vi "Module (Top Level).vi"(8 "error in":errorcluster) -> (0 "error out":errorcluster)   [LabVIEW 2017, in "Error Handler.lvlib"]
uses:
  Error Handler.lvlib
  User Events/TypeDefs/Shutdown UE FGV Command.ctl
  Global TypeDefs/Registered Modules.ctl
  <vilib>/Utility/error.llb/DialogType.ctl
  mypam/Public TypeDefs/Module Events.ctl
  Game/Public TypeDefs/Module Events.ctl
  winhost/Public TypeDefs/Module Events.ctl
  Private TypeDefs/Messages.ctl
  Logger/Logger.lvlib
  Controller/Controller.lvlib
  Game/Game.lvlib
  WinHost/WinHost.lvlib
  mypam/myPAM.lvlib
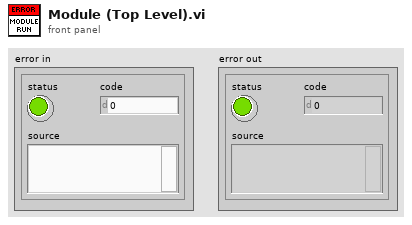
[diagram p1: front panel]
types:
  T1 = typedef "Registered Modules.ctl" = enum16{"Controller", "DAQ", "Error Handler", "Game", "myPAM", "WinHost", "Logger"}
  T2 = typedef "Shutdown UE FGV Command.ctl" = enum16{"create", "get", "destroy"}
  T3 = typedef "Controller.lvlib/Module Reference.ctl" = cluster{"calling module":T1, "module queues":T4, "module notifiers":T5}
  T4 = typedef "Controller.lvlib/Module Queues.ctl" = cluster{"message queue":refnum<queue>}
  T5 = typedef "Controller.lvlib/Module Notifiers.ctl" = cluster{"dummy notifier":refnum<notifier>}
  T6 = typedef "Logger.lvlib/Module Reference.ctl" = cluster{"calling module":T1, "module queues":T7, "module notifiers":T8}
  T7 = typedef "Logger.lvlib/Module Queues.ctl" = cluster{"message queue":refnum<queue>}
  T8 = typedef "Logger.lvlib/Module Notifiers.ctl" = cluster{"dummy notifier":refnum<notifier>}
  T9 = typedef "Error Handler.lvlib/Module Reference.ctl" = cluster{"calling module":T1, "module queues":T10, "module notifiers":T11}
  T10 = typedef "Error Handler.lvlib/Module Queues.ctl" = cluster{"message queue":refnum<queue>}
  T11 = typedef "Error Handler.lvlib/Module Notifiers.ctl" = cluster{"dummy notifier":refnum<notifier>}
  T12 = typedef "myPAM.lvlib/Module Events.ctl" = enum16{"critical error"}
  T13 = typedef "Game.lvlib/Module Events.ctl" = enum16{"client connected", "client status change", "client disconnected"}
  T14 = typedef "WinHost.lvlib/Module Events.ctl" = enum16{"host connected", "enable assistance", "disable assistance", "host disconnected"}
  T15 = typedef "Error Handler.lvlib/Messages.ctl" = enum16{"handle error", "shutdown"}
  T16 = typedef "DialogType.ctl" = u16
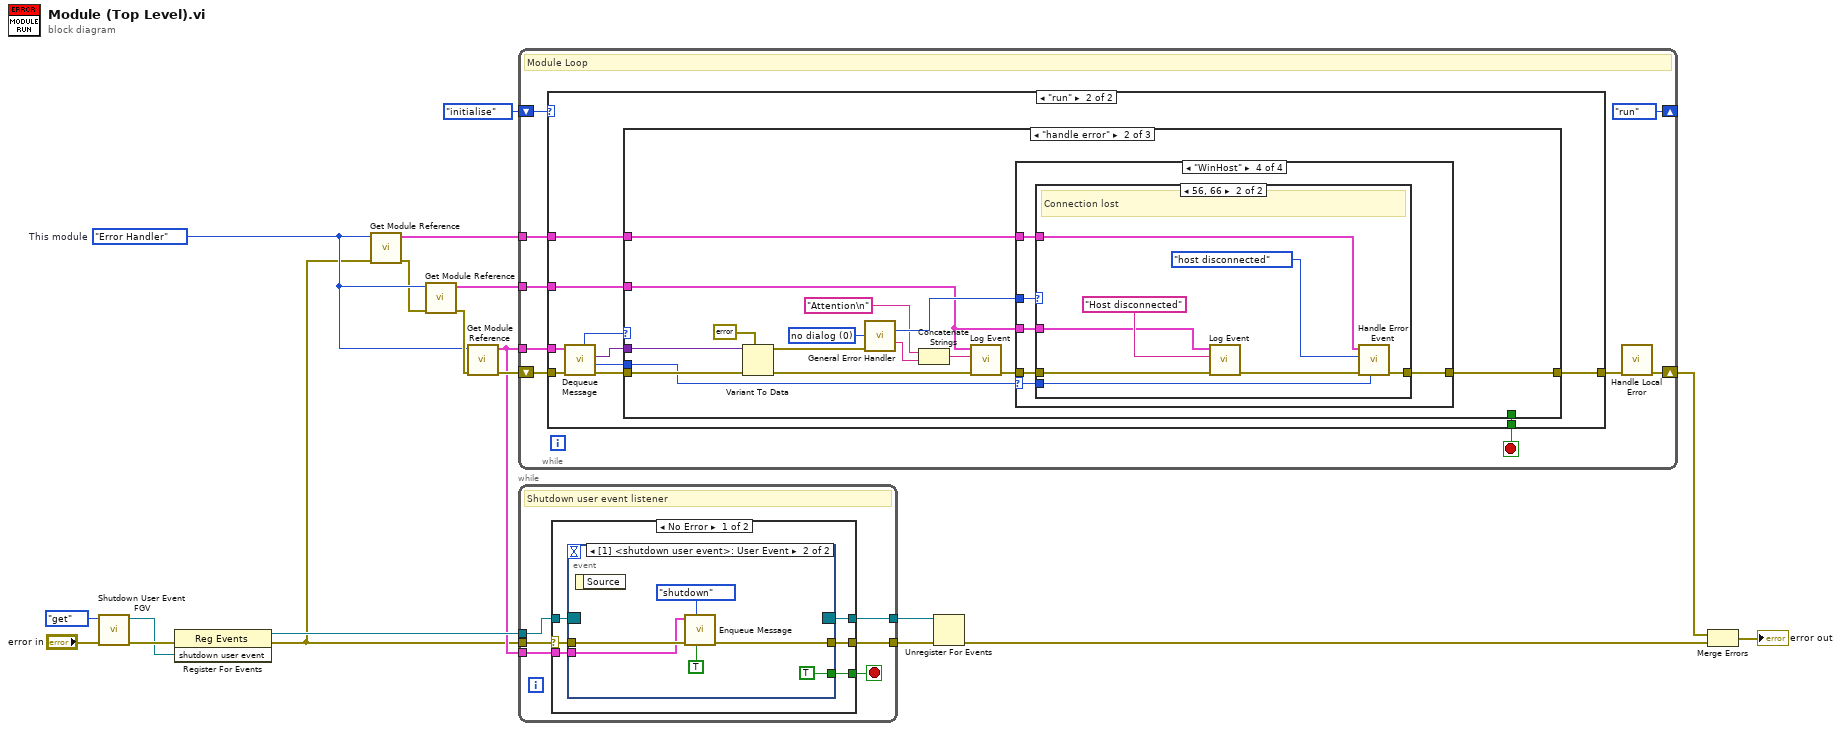
[diagram p0: block diagram]
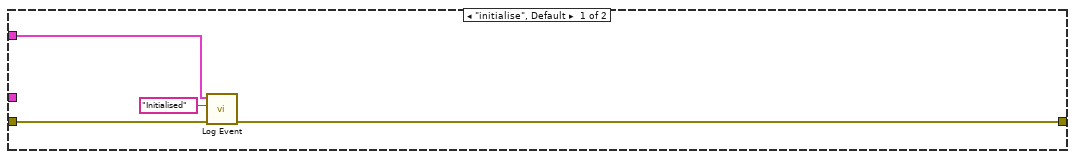
[diagram p2: hidden frame]
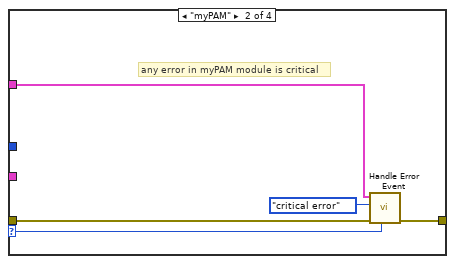
[diagram p5: hidden frame]
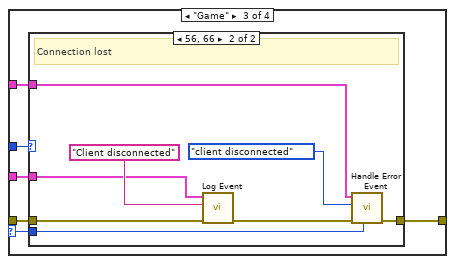
[diagram p6: hidden frame]
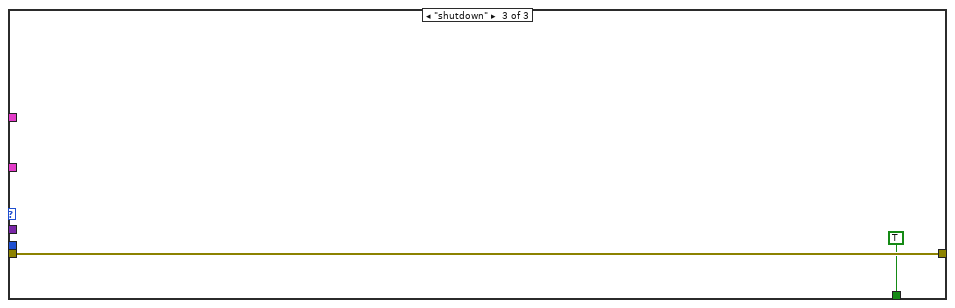
[diagram p9: hidden frame]
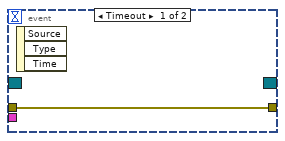
[diagram p10: hidden frame]
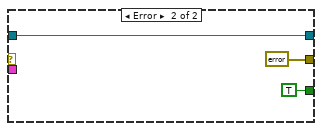
[diagram p11: hidden frame]
diagram:
  w4 = Registered_Modules."Error Handler"  # This module
  n1 = call "Shutdown User Event FGV.vi"("error in"="error in", "command"=Shutdown_UE_FGV_Command."get" ("Command")) -> ("error out"=w14:errorcluster, "shutdown user event"=w13:refnum<user-event>)  [unwired: 8 in]
  n2 = register-events(error in=w14, w13) -> (reference out=w18:refnum<event-registration>, error out=w3:errorcluster)  [unwired: 1 in]
  n3 = call "Get Module Reference.vi"("error in"=w3, "calling module"=w4) -> ("error out"=w2:errorcluster, "module reference"=w1:T3)  [unwired: 8 in]
  n4 = call "Get Module Reference.vi"("error in"=w2, "calling module"=w4) -> ("error out"=w6:errorcluster, "module reference"=w5:T6)  [unwired: 8 in]
  n5 = call "Get Module Reference.vi"("error in"=w6, "calling module"=w4) -> ("error out"=w10:errorcluster, "module reference"=w9:T9)  [unwired: 8 in]
  n6 = while {
    shift-right: [w21] -> w16
    shift-left: w10 -> [w24]
    tunnel: w9 -> [w28]
    shift-right: [enum16{"initialise", "run"}."run"] -> _
    shift-left: enum16{"initialise", "run"}."initialise" -> [w27]
    tunnel: w5 -> [w23]
    tunnel: w1 -> [w20]
    stop <- w25 stop-if-true
    # "Module Loop"
    n7 = case shown="\"run\"" w27 {
      tunnel: [w30 w42] -> w22
      tunnel: w28 -> [_ w41]
      tunnel: [_ w36] -> w25
      tunnel: w24 -> [w31 w35]
      tunnel: w23 -> [w29 w34]
      tunnel: w20 -> [_ w33]
      frame "initialise", Default {
        n8 = call "Log Event.vi"("error in"=w31, "event"="Initialised" ("string"), "module reference in"=w29) -> ("error out"=w30:errorcluster)  [unwired: 7 in, 1 out]
      }
      frame "run" {
        n9 = call "Dequeue Message.vi"("error in"=w35, "module reference in"=w41) -> ("error out"=w39:errorcluster, "source"=w37:T1, "data"=w38:variant, "message"=w40:T15)  [unwired: 5 in, 1 out]
        n10 = case shown="\"handle error\"" w40 {
          tunnel: [w43 w47 w96] -> w42
          tunnel: w39 -> [w43 w52 w96]
          tunnel: w38 -> [_ w45 _]
          tunnel: w37 -> [_ w51 _]
          tunnel: [_ _ TRUE] -> w36
          tunnel: w34 -> [_ w46 _]
          tunnel: w33 -> [_ w44 _]
          frame Default {
          }
          frame "handle error" {
            w56 = T16 0 items=["no dialog", "OK message", "continue or stop message", "OK message + warnings", "continue/stop + warnings"] ("type of dialog (OK msg:1)")
            n11 = Variant To Data(error in=w52, type=errorcluster {"status"=FALSE, "code"=0, "source"=""} ("error constant"), Variant=w45) -> (data=w57:errorcluster, error out=w50:errorcluster)
            n12 = call <vilib>:"General Error Handler.vi"("type of dialog (OK msg:1)"=w56, "error in (no error)"=w57) -> ("code out"=w55:i32, "message"=w53:string)  [unwired: 9 in, 3 out]
            n13 = Concatenate Strings("Attention\n" ("string"), w53) -> (w48:string)
            n14 = call "Log Event.vi"("error in"=w50, "event"=w48, "module reference in"=w46) -> ("error out"=w49:errorcluster)  [unwired: 7 in, 1 out]
            n15 = case shown="\"WinHost\"" w51 {
              selector: w51 -> [_ w60 w67 w82]
              tunnel: w55 -> [_ _ w70 w85]
              tunnel: w49 -> [w59 w63 w69 w84]
              tunnel: [w59 w62 w68 w83] -> w47
              tunnel: w46 -> [_ _ w66 w81]
              tunnel: w44 -> [_ w61 w65 w80]
              frame Default {
              }
              frame "myPAM" {
                # "any error in myPAM module is critical"
                n16 = call "Handle Error Event.vi"("error source"=w60, "error in"=w63, "event"=Module_Events."critical error" ("module events"), "module reference in"=w61) -> ("error out"=w62:errorcluster)  [unwired: 6 in, 1 out]
              }
              frame "Game" {
                n17 = case shown="56, 66" w70 {
                  tunnel: w69 -> [w71 w79]
                  tunnel: [w71 w74] -> w68
                  tunnel: w67 -> [_ w75]
                  tunnel: w66 -> [_ w77]
                  tunnel: w65 -> [_ w73]
                  frame Default {
                  }
                  frame 56, 66 {
                    # "Connection lost"
                    n18 = call "Log Event.vi"("error in"=w79, "event"="Client disconnected", "module reference in"=w77) -> ("error out"=w76:errorcluster)  [unwired: 7 in, 1 out]
                    n19 = call "Handle Error Event.vi"("error source"=w75, "error in"=w76, "event"=Module_Events."client disconnected" ("module events"), "module reference in"=w73) -> ("error out"=w74:errorcluster)  [unwired: 6 in, 1 out]
                  }
                }
              }
              frame "WinHost" {
                n20 = case shown="56, 66" w85 {
                  tunnel: w84 -> [w86 w94]
                  tunnel: [w86 w89] -> w83
                  tunnel: w82 -> [_ w90]
                  tunnel: w81 -> [_ w92]
                  tunnel: w80 -> [_ w88]
                  frame Default {
                  }
                  frame 56, 66 {
                    # "Connection lost"
                    n21 = call "Log Event.vi"("error in"=w94, "event"="Host disconnected", "module reference in"=w92) -> ("error out"=w91:errorcluster)  [unwired: 7 in, 1 out]
                    n22 = call "Handle Error Event.vi"("error source"=w90, "error in"=w91, "event"=Module_Events."host disconnected" ("module events"), "module reference in"=w88) -> ("error out"=w89:errorcluster)  [unwired: 6 in, 1 out]
                  }
                }
              }
            }
          }
          frame "shutdown" {
          }
        }
      }
    }
    n23 = call "Handle Local Error.vi"("error in"=w22) -> ("error out"=w21:errorcluster)  [unwired: 10 in]
  }
  n24 = while {
    tunnel: w18 -> [w102]
    tunnel: [w101] -> w17
    tunnel: w3 -> [w99]
    tunnel: [w98] -> w12
    tunnel: w9 -> [w97]
    stop <- w100 stop-if-true
    # "Shutdown user event listener"
    n25 = case shown="No Error" w99 {
      selector: w99 -> [w105 _]
      tunnel: w102 -> [w108 w117]
      tunnel: [w107 w117] -> w101
      tunnel: [w106 TRUE] -> w100
      tunnel: [w104 errorcluster {"status"=FALSE, "code"=0, "source"=""} ("error out")] -> w98
      tunnel: w97 -> [w103 _]
      frame No Error {
        n26 = event shown="[1] <shutdown user event>: User Event" {
          selector: w108 -> [_ _]
          dyn-events: [_ _] -> w107
          timeout: _ -> [_ _]
          tunnel: w105 -> [w109 w113]
          tunnel: [w109 w112] -> w104
          tunnel: [_ TRUE] -> w106
          tunnel: w103 -> [_ w111]
          event Timeout {
            n27 = event-data() -> ()  [unwired: 1 in, 3 out]
          }
          event User Event {
            n28 = event-data() -> ()  [unwired: 1 in, 1 out]
            n29 = call "Enqueue Message.vi"("high priority"=TRUE, "message"=Messages."shutdown", "error in"=w113, "module reference in"=w111) -> ("error out"=w112:errorcluster)  [unwired: 6 in, 1 out]
          }
        }
      }
      frame Error {
      }
    }
  }
  n30 = Unregister For Events(event registration refnum=w17, error in=w12) -> (error out=w7:errorcluster)
  n31 = Merge Errors(w16, w7) -> (→"error out":errorcluster)
